vi "Valid_Extra_Command.vi"(0 "Extra Commands string":string, 1 "Valid Commands Array":string[](array[string])) -> (5 "Output String":string, 6 "Extra Commands string Out":string)   [LabVIEW 2021]
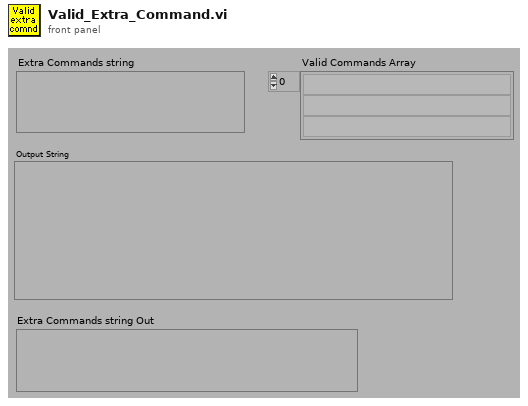
[diagram p1: front panel]
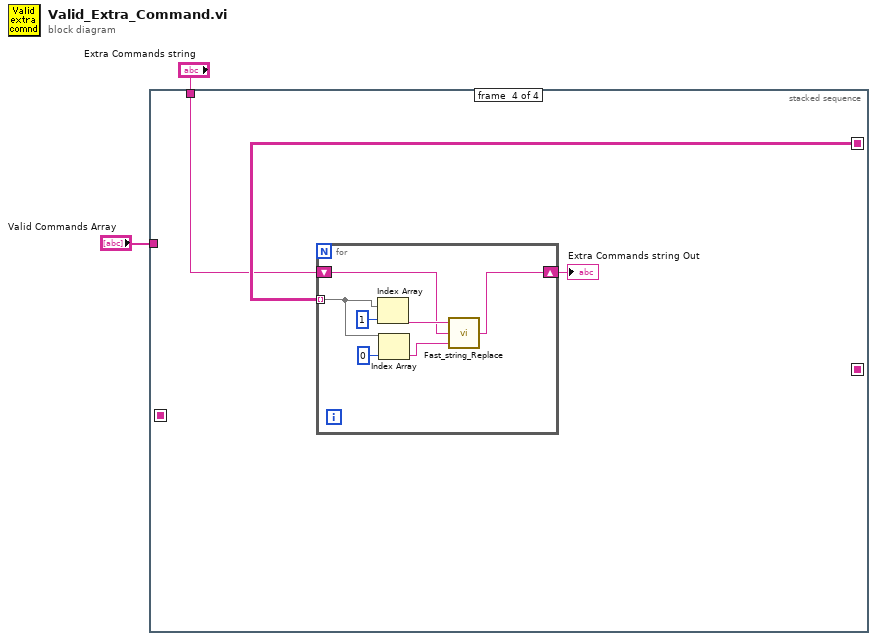
[diagram p0: block diagram]
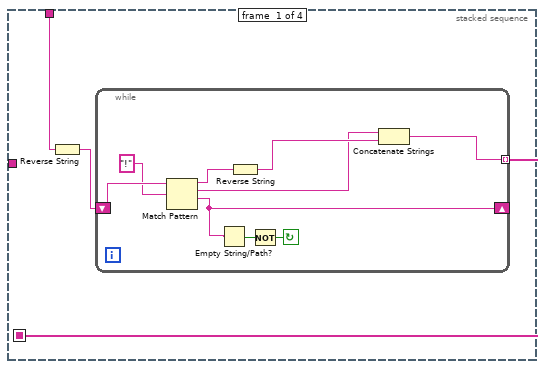
[diagram p2: hidden frame]
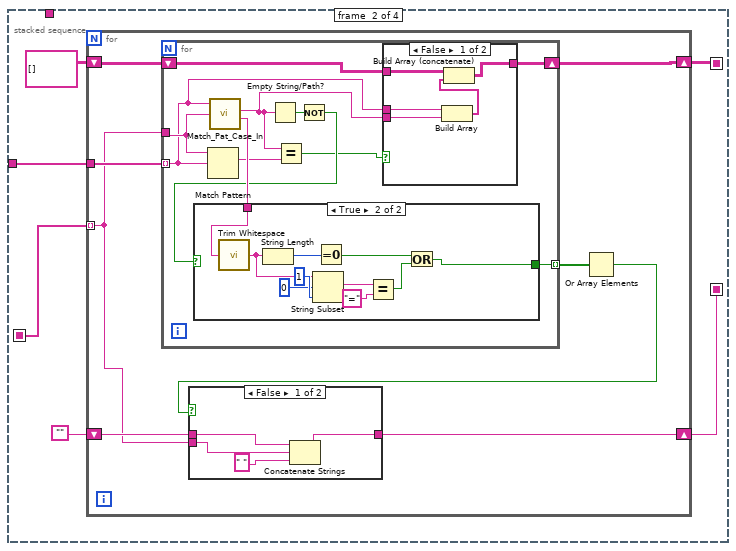
[diagram p3: hidden frame]
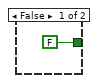
[diagram p6: hidden frame]
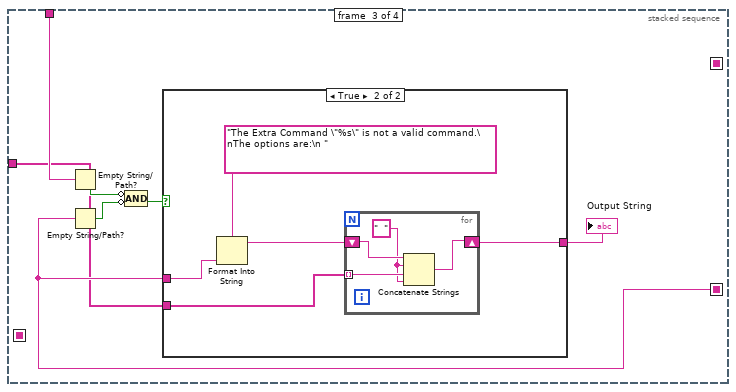
[diagram p7: hidden frame]
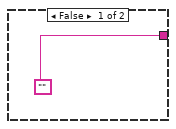
[diagram p8: hidden frame]
diagram:
  n1 = stacked-sequence {
    seq-local: [w3 _ _ _] -> [_ w20 _ _]
    seq-local: [_ w19 _ _] -> [_ _ w68 _]
    seq-local: [_ w15 _ _] -> [_ _ _ w81]
    tunnel: "Valid Commands Array" -> [_ w17 w62 _]
    tunnel: "Extra Commands string" -> [w4 _ w67 w80]
    frame #0 {
      n2 = Reverse String(1:w4) -> (0:w5:string)
      n3 = while {
        tunnel: [w10] -> w3 mode=indexing
        shift-left: w5 -> [w13]
        shift-right: [w9] -> _
        stop <- w14 continue-if-true
        n4 = Match Pattern(string=w13, regular expression="!") -> (before substring=w12:string, match substring=w6:string, after substring=w9:string)  [unwired: 2 out]
        n5 = Empty String/Path?(string/path=w9) -> (empty?=w8:bool)
        n6 = Reverse String(1:w12) -> (0:w11:string)
        n7 = Not(x=w8) -> (.not. x?=w14:bool)
        n8 = Concatenate Strings(w6, w11) -> (w10:string)
      }
    }
    frame #1 {
      n9 = for {
        tunnel: w17 -> [w28]
        tunnel: w20 -> [w23] mode=indexing
        shift-right: [w24] -> w19
        shift-left: "" -> [w25]
        shift-right: [w21] -> w15
        shift-left: string[][] [] -> [w22]
        n10 = for {
          tunnel: w28 -> [w38] mode=indexing
          tunnel: w23 -> [w43]
          tunnel: [w44] -> w27 mode=indexing
          shift-right: [w34] -> w21
          shift-left: w22 -> [w35]
          n11 = Match Pattern(string=w43, regular expression=w38) -> (match substring=w39:string)  [unwired: 4 out]
          n12 = call "Match_Pat_Case_In.vi"("String to match"=w38, "String"=w43) -> ("Matched string"=w37:string, "After  Matched string"=w41:string)  [unwired: 1 in, 2 out]
          n13 = Empty String/Path?(string/path=w37) -> (empty?=w42:bool)
          n14 = Equal?(x=w37, y=w39) -> (x = y?=w36:bool)
          n15 = Not(x=w42) -> (.not. x?=w40:bool)
          n16 = case shown="True" w40 {
            tunnel: w41 -> [_ w61]
            tunnel: [FALSE w52] -> w44
            frame False {
            }
            frame True {
              n17 = call <vilib>:"Trim Whitespace.vi"("string"=w61) -> ("trimmed string"=w58:string)  [unwired: 1 in]
              n18 = String Length(string=w58) -> (length=w55:i32)
              n19 = String Subset(string=w58, offset (0)=0, length (rest)=1 ("length")) -> (substring=w57:string)
              n20 = Equal To 0?(x=w55) -> (x = 0?=w54:bool)
              n21 = Equal?(x=w57, y="=") -> (x = y?=w53:bool)
              n22 = Or(x=w54, y=w53) -> (x .or. y?=w52:bool)
            }
          }
          n23 = case shown="False" w36 {
            tunnel: w38 -> [w49 _]
            tunnel: w37 -> [w48 _]
            tunnel: w35 -> [w46 w50]
            tunnel: [w45 w50] -> w34
            frame False {
              n24 = Build Array(w49, w48) -> (w47:string[])
              n25 = Build Array (concatenate)(w46, w47) -> (w45:string[][])
            }
            frame True {
            }
          }
        }
        n26 = Or Array Elements(Boolean array=w27) -> (logical OR=w26:bool)
        n27 = case shown="False" w26 {
          tunnel: w25 -> [w29 w33]
          tunnel: w23 -> [w31 _]
          tunnel: [w32 w33] -> w24
          frame False {
            n28 = Concatenate Strings(w29, w31, " ") -> (w32:string)
          }
          frame True {
          }
        }
      }
    }
    frame #2 {
      n29 = Empty String/Path?(string/path=w67) -> (empty?=w65:bool)
      n30 = Empty String/Path?(string/path=w68) -> (empty?=w66:bool)
      n31 = Compound Arithmetic op=AND(invert w65, invert w66) -> (w64:bool)
      n32 = case shown="True" w64 {
        tunnel: w68 -> [_ w74]
        tunnel: ["" w70] -> w63
        tunnel: w62 -> [_ w71]
        frame False {
        }
        frame True {
          n33 = Format Into String(format string="The Extra Command \"%s\" is not a valid command.\nThe options are:\n " ("Format String"), w74) -> (resulting string=w72:string)  [unwired: 2 in, 1 out]
          n34 = for {
            shift-right: [w76] -> w70
            shift-left: w72 -> [w77]
            tunnel: w71 -> [w78] mode=indexing
            w75 = "  " ("Substring")
            n35 = Concatenate Strings(w77, w75, w78, w75) -> (w76:string)
          }
        }
      }
      "Output String" <- w63
    }
    frame #3 {
      n36 = for {
        tunnel: w81 -> [w86] mode=indexing
        shift-right: [w83] -> w79
        shift-left: w80 -> [w84]
        n37 = Index Array(array=w86, index=1) -> (element=w85:string)
        n38 = Index Array(array=w86, index=0) -> (element=w82:string)
        n39 = call "Fast_string_Replace.vi"("Replace match with:"=w82, "Input String"=w84, "regular expression"=w85) -> ("Output String"=w83:string)  [unwired: 2 out]
      }
      "Extra Commands string Out" <- w79
    }
  }
